vi "Create RIO Data Files.vi"(6 "Serial Numbers":string[](array[string]), 9 "Base Filepath":path, 10 "File Index In":i32, 11 "Anomaly Filepath In":path) -> (1 "Current Filepath":path, 2 "File Index Out":i32, 3 "Anomaly Filepath Out":path)   [LabVIEW 2019]
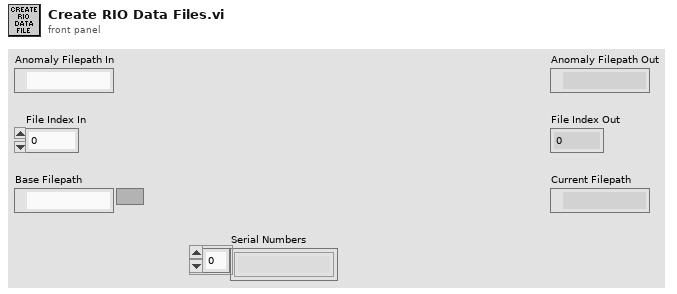
[diagram p1: front panel]
types:
  T1 = enum16{"open", "replace", "create", "open or create", "replace or create", "replace or create with confirmation"}
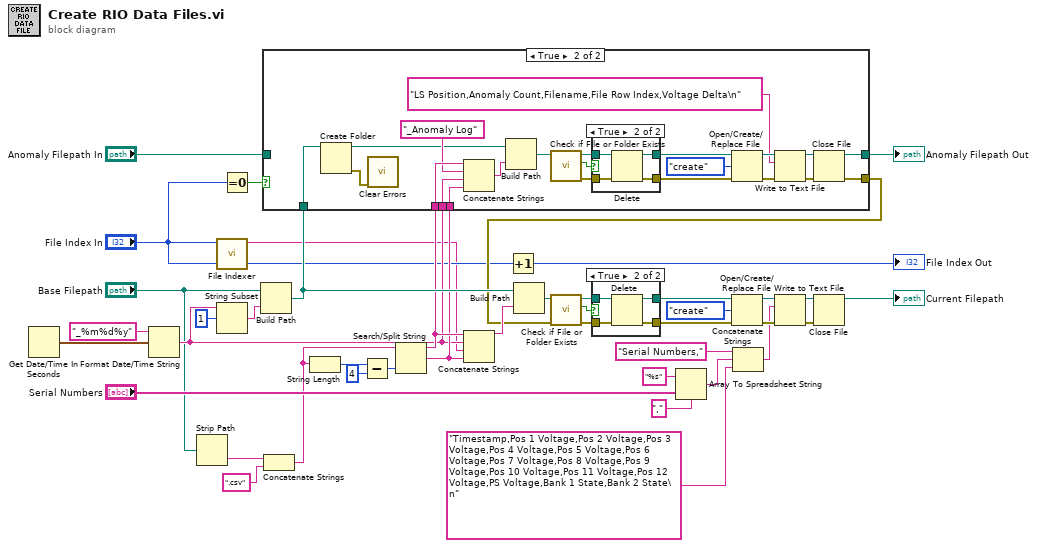
[diagram p0: block diagram]
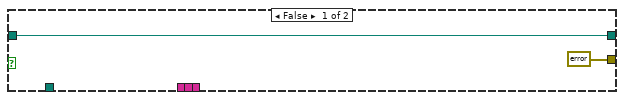
[diagram p2: hidden frame]
diagram:
  n1 = Get Date/Time In Seconds() -> (seconds since 1Jan1904=w20:timestamp)
  n2 = Format Date/Time String(time format string (%c)="_%m%d%y", seconds (now)=w20) -> (date/time string=w11:string)  [unwired: 1 in]
  n3 = Strip Path(path="Base Filepath") -> (name=w6:string)  [unwired: 1 out]
  n4 = call "File Indexer.vi"("File Index In"="File Index In") -> ("File Indicator Out"=w2:string)  [unwired: 10 in]
  n5 = String Subset(string=w11, offset (0)=1) -> (substring=w10:string)  [unwired: 1 in]
  n6 = Equal To 0?(x="File Index In") -> (x = 0?=w13:bool)
  n7 = Build Path(base path="Base Filepath", name or relative path=w10) -> (appended path=w17:path)
  n8 = Concatenate Strings(w6, ".csv" ("string")) -> (w4:string)
  n9 = String Length(string=w4) -> (length=w23:i32)
  n10 = Subtract(x=w23, y=4) -> (x-y=w21:i32)
  n11 = Search/Split String(string=w4, offset (0)=w21) -> (substring before match=w16:string, match + rest of string=w15:string)  [unwired: 1 in, 1 out]
  n12 = case shown="True" w13 {
    tunnel: w17 -> [_ w47]
    tunnel: w16 -> [_ w65]
    tunnel: w15 -> [_ w64]
    tunnel: w11 -> [_ w63]
    tunnel: [w44 w61] -> w14
    tunnel: "Anomaly Filepath In" -> [w44 _]
    tunnel: [errorcluster {"status"=FALSE, "code"=0, "source"=""} ("error out") w48] -> w8
    frame False {
    }
    frame True {
      n13 = Create Folder(path (use dialog)=w47) -> (created path=w46:path, error out=w45:errorcluster)  [unwired: 2 in, 1 out]
      n14 = call <vilib>:"Clear Errors.vi"("error in (no error)"=w45) -> ()  [unwired: 5 in, 2 out]
      n15 = Concatenate Strings(w65, "_Anomaly Log" ("string"), w63, w64) -> (w66:string)
      n16 = Build Path(base path=w46, name or relative path=w66) -> (appended path=w50:path)
      n17 = call <vilib>:"Check if File or Folder Exists.vi"("path"=w50) -> ("error out"=w52:errorcluster, "file or folder exists?"=w60:bool, "dup path"=w59:path)  [unwired: 8 in]
      n18 = case shown="True" w60 {
        tunnel: w59 -> [w68 w72]
        tunnel: [w68 w71] -> w53
        tunnel: w52 -> [w67 w70]
        tunnel: [w67 w69] -> w51
        frame False {
        }
        frame True {
          n19 = Delete(path (use dialog)=w72, error in=w70) -> (deleted path=w71:path, error out=w69:errorcluster)  [unwired: 3 in, 1 out]
        }
      }
      n20 = Open/Create/Replace File(file path (use dialog)=w53, error in=w51, operation (0:open)=T1."create") -> (refnum out=w57:refnum<file>, error out=w55:errorcluster)  [unwired: 3 in, 1 out]
      n21 = Write to Text File(file (use dialog)=w57, text="LS Position,Anomaly Count,Filename,File Row Index,Voltage Delta\n", error in=w55) -> (refnum out=w58:refnum<file>, error out=w56:errorcluster)  [unwired: 1 in, 1 out]
      n22 = Close File(refnum=w58, error in=w56) -> (path=w61:path, error out=w48:errorcluster)
    }
  }
  "Anomaly Filepath Out" <- w14
  n23 = Concatenate Strings(w16, w11, w2, w15) -> (w18:string)
  n24 = Increment(x="File Index In") -> (x+1=→"File Index Out":i32)
  n25 = Build Path(base path=w17, name or relative path=w18) -> (appended path=w27:path)
  n26 = call <vilib>:"Check if File or Folder Exists.vi"("error in (no error)"=w8, "path"=w27) -> ("error out"=w41:errorcluster, "file or folder exists?"=w28:bool, "dup path"=w29:path)  [unwired: 7 in]
  n27 = case shown="True" w28 {
    tunnel: w29 -> [w74 w78]
    tunnel: [w74 w77] -> w40
    tunnel: w41 -> [w73 w76]
    tunnel: [w73 w75] -> w42
    frame False {
    }
    frame True {
      n28 = Delete(path (use dialog)=w78, error in=w76) -> (deleted path=w77:path, error out=w75:errorcluster)  [unwired: 3 in, 1 out]
    }
  }
  n29 = Array To Spreadsheet String(delimiter (Tab)=",", array="Serial Numbers", 3:"%s" ("format string")) -> (spreadsheet string=w30:string)
  n30 = Open/Create/Replace File(file path (use dialog)=w40, error in=w42, operation (0:open)=T1."create") -> (refnum out=w36:refnum<file>, error out=w38:errorcluster)  [unwired: 3 in, 1 out]
  n31 = Concatenate Strings("Serial Numbers," ("string"), w30, "Timestamp,Pos 1 Voltage,Pos 2 Voltage,Pos 3 Voltage,Pos 4 Voltage,Pos 5 Voltage,Pos 6 Voltage,Pos 7 Voltage,Pos 8 Voltage,Pos 9 Voltage,Pos 10 Voltage,Pos 11 Voltage,Pos 12 Voltage,PS Voltage,Bank 1 State,Bank 2 State\n") -> (w33:string)
  n32 = Write to Text File(file (use dialog)=w36, text=w33, error in=w38) -> (refnum out=w35:refnum<file>, error out=w37:errorcluster)  [unwired: 1 in, 1 out]
  n33 = Close File(refnum=w35, error in=w37) -> (path=→"Current Filepath":path)  [unwired: 1 out]
